vi "Read Heater.vi"(11 "Freezer in":refnum<class "Freezer.lvclass">) -> (2 "Blower/Heater":T1, 3 "Freezer out":refnum<class "Freezer.lvclass">)   [LabVIEW 2015, in "cRIO-Carbondioxide.lvlib" / "CO2-Actor.lvlib" / "Freezer.lvclass"]
uses:
  Freezer.lvclass
  cRIO-CO2/Blowers Heaters Enumerator.ctl
  Freezer.lvclass/Freezer.ctl
  cRIO-CO2/cRIO-CO2.lvclass
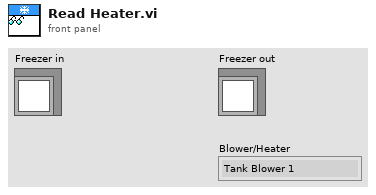
[diagram p1: front panel]
types:
  T1 = typedef "cRIO-Carbondioxide.lvlib/cRIO-CO2.lvlib/cRIO-CO2.lvclass/Blowers Heaters Enumerator.ctl" = enum16{"Tank Blower 1", "Tank Blower 2", "Tank Blower 3", "Tank Blower 4", "Syringe Blower", "Syringe Heater", "Piston Heater", "Undefined"}
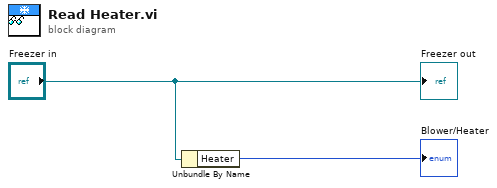
[diagram p0: block diagram]
diagram:
  n1 = Unbundle By Name("Freezer in") -> ("Heater"=→"Blower/Heater":T1)
  "Freezer out" <- "Freezer in"
